vi "SPI MOSI.vi"(7 "Index":T1, 8 "Setup?":bool, 9 "LSB first?":bool, 10 "Load?":bool, 11 "Data Out":u16) -> (3 "MOSI":bool)   [LabVIEW 2019]
uses:
  SPI Frame Length.ctl
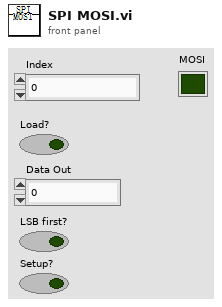
[diagram p1: front panel]
types:
  T1 = typedef "SPI Frame Length.ctl" = fxp<+,4,4>
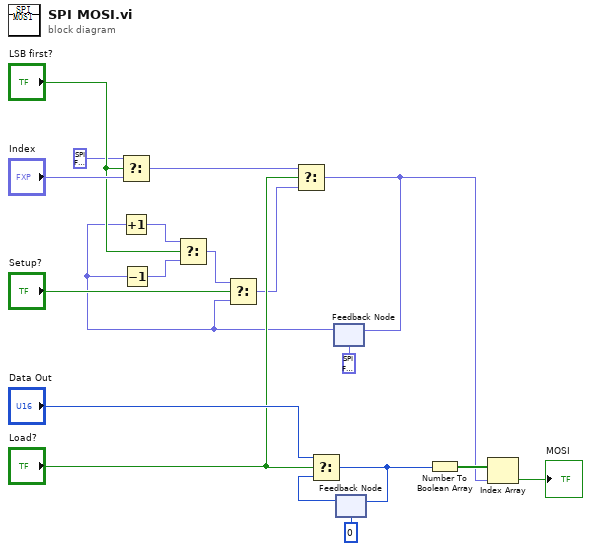
[diagram p0: block diagram]
diagram:
  n1 = Select(t=T1 0.0, s="LSB first?", f="Index") -> (s? t:f=w3:T1)
  n2 = feedback #1(T1 0.0 ("Index")) -> (w2:T1)
  n3 = Increment(x=w2) -> (x+1=w8:T1)
  n4 = Decrement(x=w2) -> (x-1=w7:T1)
  n5 = Select(t=w8, s="LSB first?", f=w7) -> (s? t:f=w6:T1)
  n6 = Select(t=w6, s="Setup?", f=w2) -> (s? t:f=w5:T1)
  n7 = Select(t=w3, s="Load?", f=w5) -> (s? t:f=w1:T1)
  n8 = feedback-in #1(w1) -> ()
  n9 = feedback #2(u16 0 ("Data Out")) -> (w16:u16)
  n10 = Select(t="Data Out", s="Load?", f=w16) -> (s? t:f=w12:u16)
  n11 = feedback-in #2(w12) -> ()
  n12 = Number To Boolean Array(number=w12) -> (Boolean array=w18:bool[])
  n13 = Index Array(array=w18, index=w1) -> (element=→"MOSI":bool)
